vi "LinTest.vi"() -> ()   [LabVIEW 2018]
uses:
  Crl/LIN_DataType.ctl
panel:
  in  "hold log?":bool
  in  "Program":string
  in  "Config":bool
  out "错误输出":errorcluster
  in  "NAD":u8 format="%.0x"
  in  "LDF filepath":path
  in  "interface":refnum<k21>="LIN1"
  in  "Seq?":bool
  in  "EXIT":bool
  in  "Send Data":T1=[{"send?"=FALSE, "payload"=[3, 34, 241, 80, 0, 0, 0, 0], "Delays"=200, "Note"="软件版本", "mult?"=FALSE, "Seq"=0}, {"send?"=FALSE, "payload"=[3, 34, 241, 81, 0, 0, 0, 0], "Delays"=200, "Note"="硬件版本", "mult?"=FALSE, "Seq"=0}, {"send?"=FALSE, "payload"=[3, 34, 2, 0, 0, 0, 0, 0], "Delays"=200, "Note"="玻璃位置", "mult?"=FALSE, "Seq"=0}, {"send?"=FALSE, "payload"=[4, 49, 1, 3, 10, 0, 0, 0], "Delays"=200, "Note"="初始化", "mult?"=FALSE, "Seq"=0}, {"send?"=FALSE, "payload"=[5, 49, 1, 3, 2, 2, 0, 0], "Delays"=200, "Note"="玻璃开", "mult?"=FALSE, "Seq"=0}, {"send?"=FALSE, "payload"=[4, 46, 254, 17, 4, 0, 0, 0], "Delays"=200, "Note"="设置工厂模式", "mult?"=FALSE, "Seq"=0}] {"payload" format="%02x"}
  out "Frames":string[][](table)
  in  "Send":bool
  # "Lin Test Panel"
  # "ms"
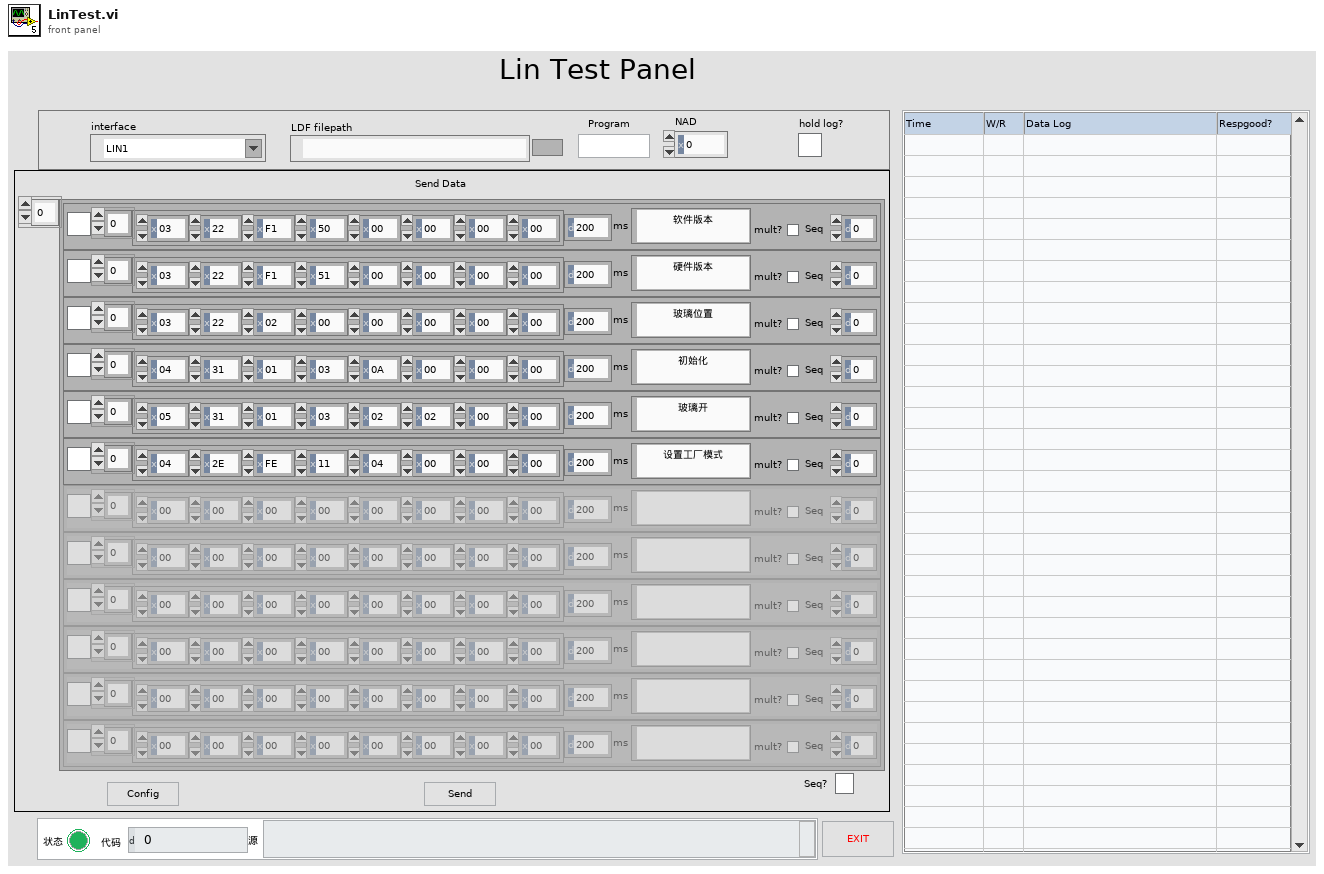
[diagram p1: front panel]
types:
  T1 = typedef "LIN_DataType.ctl" = cluster{"send?":bool, "payload":u8[], "Delays":u32, "Note":string, "mult?":bool, "Seq":i32}[]
  T2 = cluster{"appended path":path, "error":errorcluster, "Send Data":refnum<vi>, "NAD":u8}
  T3 = typedef "LIN Device.ctl" = cluster{"Master Frame(3C)":refnum<k21>, "Slave Frame(3D)":refnum<k21>, "Request Schedule":refnum<k21>, "Response Schedule":refnum<k21>, "Frame Write SCU":refnum<k21>, "Frame Read SCU":refnum<k21>, "LIN Name":refnum<k21>}
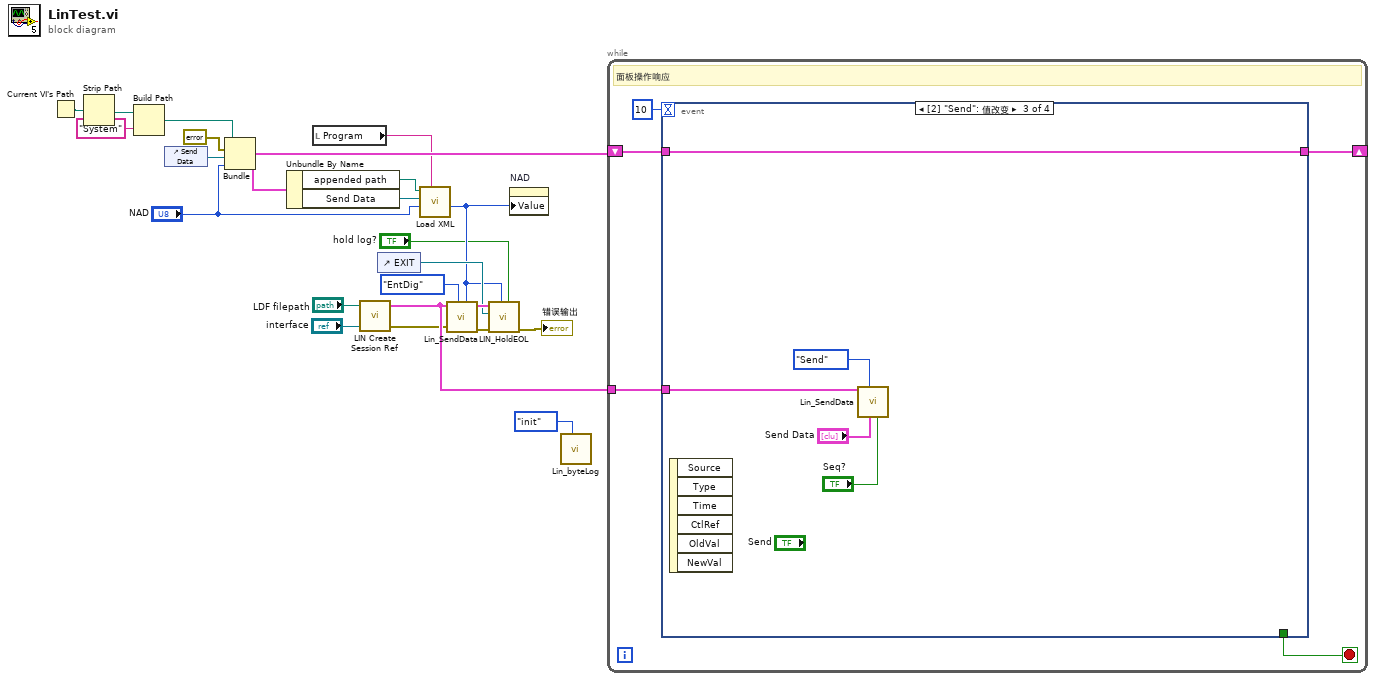
[diagram p0: block diagram]
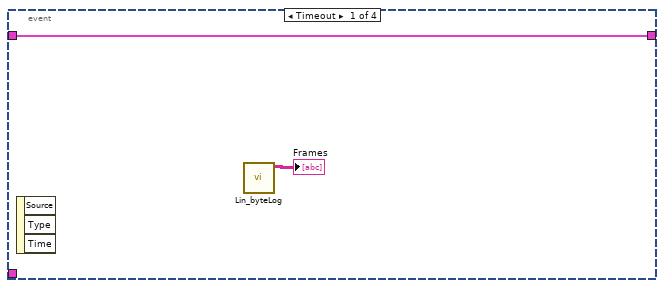
[diagram p2: hidden frame]
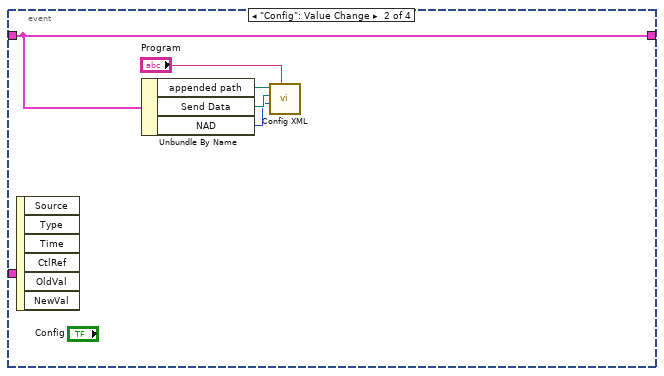
[diagram p3: hidden frame]
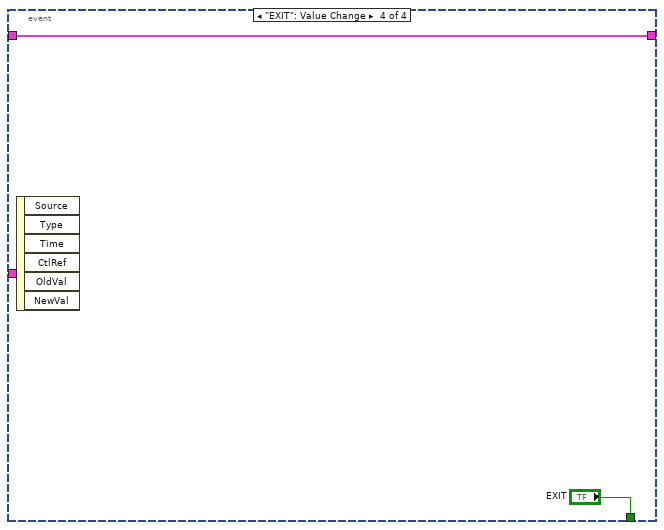
[diagram p4: hidden frame]
diagram:
  n1 = Current VI's Path() -> (path=w12:path)
  n2 = Strip Path(path=w12) -> (stripped path=w11:path)  [unwired: 1 out]
  n3 = Build Path(base path=w11, name or relative path="System" ("名称或相对路径")) -> (appended path=w9:path)
  n4 = control-ref of="Send Data"() -> (w14:refnum<vi>)
  n5 = Bundle("appended path"=w9, "error"=errorcluster {"status"=FALSE, "code"=0, "source"=""}, "Send Data"=w14, "NAD"="NAD") -> (w7:T2)  [unwired: 1 in]
  n6 = Unbundle By Name(w7) -> ("appended path"=w6:path, "Send Data"=w1:refnum<vi>)
  n7 = local read "Program"() -> (w5:string)
  n8 = call "LIN Create Session Ref.vi"("LDF filepath"="LDF filepath", "interface"="interface") -> ("LIN Device"=w22:T3, "错误输出"=w17:errorcluster)  [unwired: 5 in]
  n9 = control-ref of="EXIT"() -> (w8:refnum<vi>)
  n10 = call "Load XML.vi"("Program"=w5, "NAD"="NAD", "Send Data"=w1, "XML File Path"=w6) -> ("NAD"=w3:u8)  [unwired: 7 in]
  n11 = call "Lin_SendData.vi"("NAD"=w3, "mode"=enum16{"EntDig", "Send"}."EntDig", "Error In"=w17, "LIN Device"=w22) -> ("error IO"=w16:errorcluster, "LIN Device"=w18:T3)  [unwired: 6 in]
  n12 = call "LIN_HoldEOL.vi"("log?"="hold log?", "NAD"=w3, "Error In"=w16, "exit"=w8, "LIN Device"=w18) -> ("error IO"=→"错误输出":errorcluster)  [unwired: 6 in]
  n13 = property on="NAD" class="DigNum (严格)"("Value"=w3) -> ()  [unwired: 2 in, 2 out]
  n14 = call "Lin_byteLog.vi"("r/w"=enum16{"read", "write", "init"}."init") -> ()  [unwired: 10 in, 1 out]
  n15 = while {
    tunnel: w22 -> [w28]
    shift-right: [w26] -> _
    shift-left: w7 -> [w25]
    stop <- w24 stop-if-true
    # "面板操作响应"
    n16 = event shown="[2] \"Send\": 值改变" {
      selector: _ -> [_ _ _ _]
      dyn-events: _ -> [_ _ _ _]
      timeout: 10 -> [_ _ _ _]
      tunnel: [_ _ _ "EXIT"] -> w24
      tunnel: w28 -> [_ _ w37 _]
      tunnel: [w29 w32 w36 w42] -> w26
      tunnel: w25 -> [w29 w32 w36 w42]
      event Timeout {
        n17 = event-data() -> ()  [unwired: 1 in, 3 out]
        n18 = call "Lin_byteLog.vi"() -> ("log"=→"Frames":string[][])  [unwired: 11 in]
      }
      event "Config": Value Change {
        n19 = event-data() -> ()  [unwired: 1 in, 6 out]
        n20 = Unbundle By Name(w32) -> ("appended path"=w35:path, "Send Data"=w34:refnum<vi>, "NAD"=w31:u8)
        n21 = call "Config XML.vi"("Program"="Program", "NAD"=w31, "Send Data"=w34, "XML File Path"=w35) -> ()  [unwired: 7 in, 1 out]
      }
      event "Send": Value Change {
        n22 = event-data() -> ()  [unwired: 1 in, 6 out]
        n23 = call "Lin_SendData.vi"("Seq?"="Seq?", "Data"="Send Data", "mode"=enum16{"EntDig", "Send"}."Send", "LIN Device"=w37) -> ()  [unwired: 6 in, 2 out]
      }
      event "EXIT": Value Change {
        n24 = event-data() -> ()  [unwired: 1 in, 6 out]
      }
    }
  }
